vi "Output Stream Control.vi"(0 "start trigger":bool, 1 "reset":bool, 5 "burst size":u32, 7 "abort":bool, 9 "ready to read stream (T)":bool=TRUE, 11 "fifo output valid":bool, 12 "samples per cycle":u32=1) -> (4 "read stream":bool, 6 "state":T1, 8 "samples processed":u32, 10 "number of underflows":u32, 15 "fifo underflow":bool)   [LabVIEW 2017]
doc: "Controls whether or not data is read from the DMA FIFO for the generation stream. If burst size is 0, this will be a continuous stream, started when the start trigger is asserted. If burst size is greater than zero, generation will be in bursts of the designated size, initiated each time the internal state machine is idle and a start trigger is received.\n\nThis VI also keeps track of whether or not an underflow occurred in the generation stream and counts the number of underflows that have occurred for debugging information.\n\nThe internal state machine returns the number of samples processed since the most recent generation began and the current state machine state."
uses:
  Stream Control State.ctl
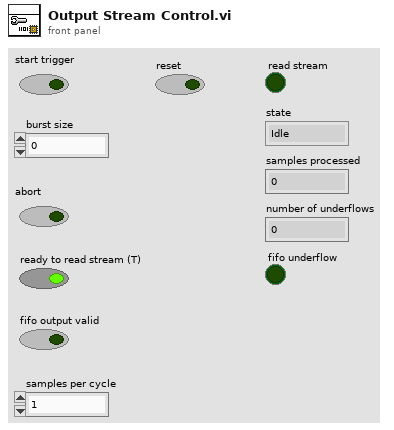
[diagram p1: front panel]
types:
  T1 = typedef "Stream Control State.ctl" = enum16{"Idle", "Active"}
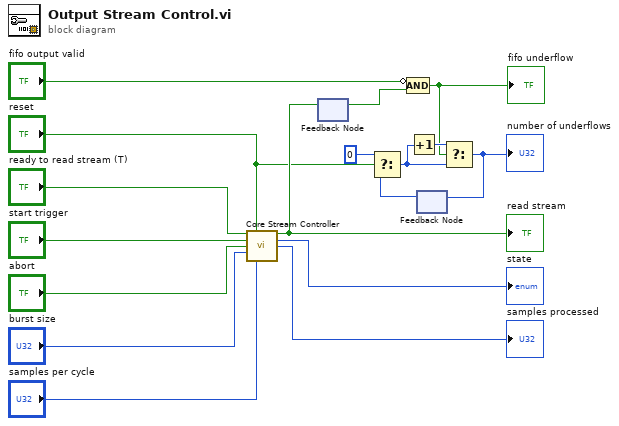
[diagram p0: block diagram]
diagram:
  n1 = call "Core Stream Controller.vi"("input valid"="ready to read stream (T)", "reset"="reset", "start trigger"="start trigger", "abort"="abort", "burst size"="burst size", "samples per cycle"="samples per cycle") -> ("write stream"=w12:bool, "state"=→"state":T1, "samples processed"=→"samples processed":u32)  [unwired: 7 in]
  "read stream" <- w12
  n2 = feedback-in #1(w12) -> ()
  n3 = feedback #1() -> (w11:bool)  [unwired: 1 in]
  n4 = Compound Arithmetic op=AND(invert "fifo output valid", w11) -> (w4:bool)
  "fifo underflow" <- w4
  n5 = feedback #2() -> (w7:u32)  [unwired: 1 in]
  n6 = Select(t=u32 0, s="reset", f=w7) -> (s? t:f=w6:u32)
  n7 = Increment(x=w6) -> (x+1=w9:u32)
  n8 = Select(t=w9, s=w4, f=w6) -> (s? t:f=w8:u32)
  "number of underflows" <- w8
  n9 = feedback-in #2(w8) -> ()
